vi "Write PLL_Configuration.vi"(8 "error in (no error)":errorcluster, 10 "Configuration":T1={"PLLgains"={"proportional gain"=0.0, "integral gain"=0.0}, "PLLrange"={"output high (Inf)"=inf, "output low (-Inf)"=-inf}, "dT"=0.0, "expectedFreq"=0.0, "lockDuration"=0.0, "freqBoundaries"=0.0, "adjustTheta"=0.0, "HarmonicFilter"={"enable"=FALSE, "coeff"={"ak"=0.0, "bk"=0.0}}} {"PLLgains"."proportional gain" step=0.125}, 11 "ThreePhasePLL configuration in":refnum<class "ThreePhasePLL configuration.lvclass">) -> (0 "error out":errorcluster, 3 "ThreePhasePLL configuration out":refnum<class "ThreePhasePLL configuration.lvclass">)   [LabVIEW 2017, in "ThreePhasePLL configuration.lvclass"]
uses:
  ThreePhasePLL configuration.lvclass
  <vilib>/NI/PowerElectronicsControl/ThreePhasePLL/Interface/Configuration.ctl
  <vilib>/rvi/Analysis/control/PID/Typedef/niFpgaPID_PIGains.ctl
  <vilib>/rvi/Analysis/control/PID/Typedef/niFpgaPID_OutputRange.ctl
  <vilib>/NI/PowerElectronicsControl/ThreePhasePLL/FPGA/HarmonicFilter.ctl
  ThreePhasePLL configuration.lvclass/ThreePhasePLL configuration.ctl
  <vilib>/NI/PowerElectronicsControl/ThreePhasePLL/Interface/ThreePhasePLLInterface.lvlib
  <vilib>/NI/PowerElectronicsControl/ThreePhasePLL/FPGA/ThreePhasePLL.lvlib
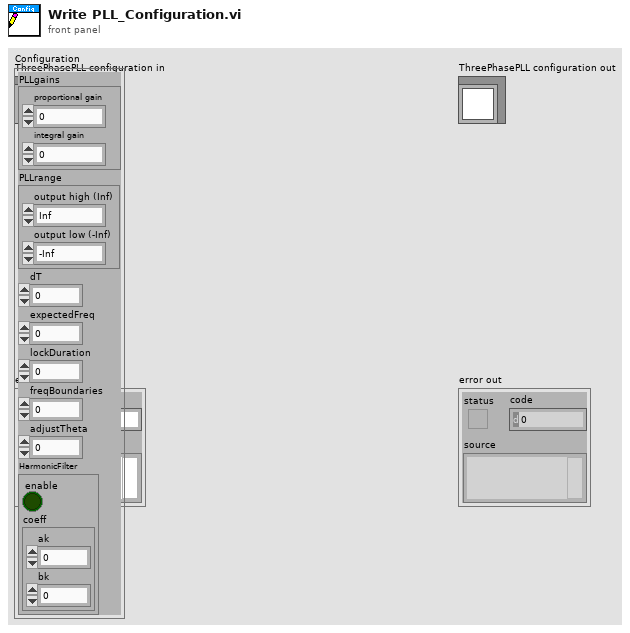
[diagram p1: front panel]
types:
  T1 = typedef "ThreePhasePLLInterface.lvlib/Configuration.ctl" = cluster{"PLLgains":T2, "PLLrange":T3, "dT":sgl, "expectedFreq":sgl, "lockDuration":sgl, "freqBoundaries":sgl, "adjustTheta":sgl, "HarmonicFilter":cluster{"enable":bool, "coeff":T4}}
  T2 = typedef "niFpgaPID_PIGains.ctl" = cluster{"proportional gain":sgl, "integral gain":sgl}
  T3 = typedef "niFpgaPID_OutputRange.ctl" = cluster{"output high (Inf)":sgl, "output low (-Inf)":sgl}
  T4 = typedef "ThreePhasePLL.lvlib/HarmonicFilter.ctl" = cluster{"ak":sgl, "bk":sgl}
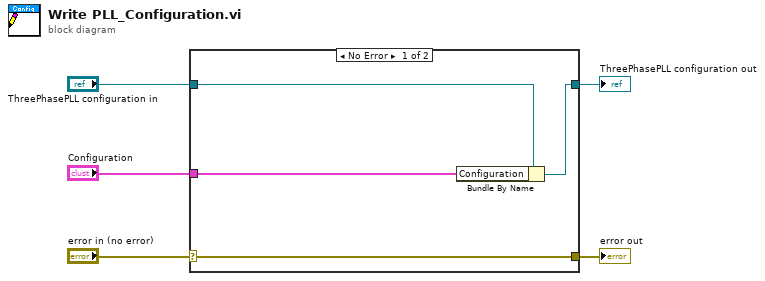
[diagram p0: block diagram]
diagram:
  n1 = case shown="No Error" "error in (no error)" {
    selector: "error in (no error)" -> [w9 w10]
    tunnel: [w9 w10] -> w4
    tunnel: [w7 w11] -> w2
    tunnel: "ThreePhasePLL configuration in" -> [w8 w11]
    tunnel: "Configuration" -> [w6 _]
    frame No Error {
      n2 = Bundle By Name(cluster=w8, "Configuration"=w6) -> (w7:refnum<class "ThreePhasePLL configuration.lvclass">)
    }
    frame Error {
    }
  }
  "error out" <- w4
  "ThreePhasePLL configuration out" <- w2
